vi "Laptop image processing Dev.vi"() -> ()   [LabVIEW 2009]
uses:
  <vilib>/userDefined/High Color/IMAQdx.ctl
  UDP Lib/UDP Network Location.ctl
  TypeDefs/cRIO-EVS Comm/EVS to cRIO UDP packet.ctl
  <vilib>/vision/driver/IMAQdx.llb/IMAQdx Acquisition Mode.ctl
  <vilib>/Platform/TimedLoop/XDataNode/XDataNode.xnode
  <vilib>/Platform/TimedLoop/XDataNode/loadlvalarms.vi
  <vilib>/Platform/TimedLoop/XDataNode/timing_clust.ctl
  <vilib>/Platform/TimedLoop/XDataNode/nitl_modes.ctl
  <vilib>/Platform/TimedLoop/XDataNode/wakeup.ctl
  <vilib>/vision/driver/NI_Vision_Acquisition_Software.lvlib
  <vilib>/Platform/TimedLoop/XDataNode/XDNodeRunTimeDep.lvlib
panel:
  out "Extracted 2":T1(plugin-control) caption="Extracted"
  out "Original 2":T1(plugin-control) caption="Original"
  out "Project:Target Item":refnum<vi>
  out "Original":T1(plugin-control)
  out "Extracted":T1(plugin-control)
  out "Ramp?":bool
  in  "Extraction mode":i32(knob) scale=0.0..2.0
  out "Iteration Duration":i64
  out "Number of ramp regions (left)":i32
  out "Number of ramp regions (right)":i32
  out "Sick array":u16[](array[numeric])
  in  "stop":bool
  out "HB":bool
  in  "IMAQdx Session Left":T2="lcam" caption="Left Session"
  in  "IMAQdx Session Right":T2="rcam" caption="Right Session"
  # "0: Original\n1: Extracted\n2: Masked"
  # "0: Old line extraction\n1: Solid white line (ramp)\n2: LPF"
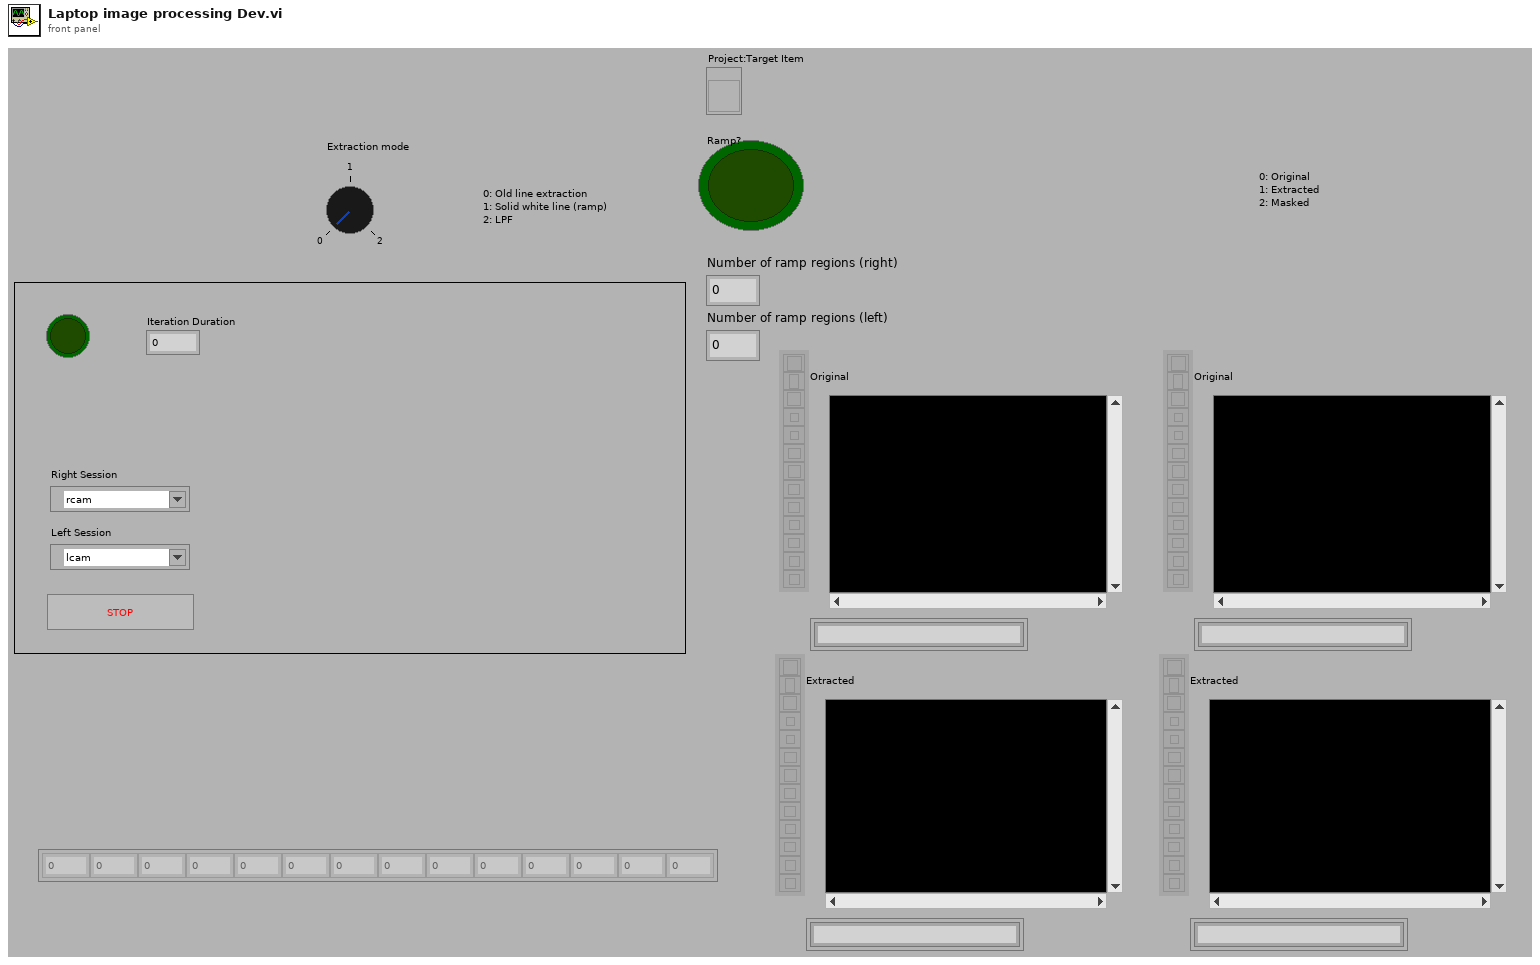
[diagram p1: front panel]
types:
  T1 = typedef "IMAQ Image.ctl" = refnum<image>
  T2 = typedef "IMAQdx.ctl" = refnum<k21>
  T3 = typedef "EVS to cRIO UDP packet.ctl" = cluster{"Camera SICK":u16[], "Camera init":bool}
  T4 = typedef "NI_Vision_Acquisition_Software.lvlib/IMAQdx Acquisition Mode.ctl" = enum32{"One Shot", "Continuous"}
  T5 = typedef "XDNodeRunTimeDep.lvlib/timing_clust.ctl" = cluster{"Expected End [f-1]":u64, "Actual End [f-1]":u64, "Finished Late? [f-1]":bool, "Expected End [i-1]":u64, "Actual End [i-1]":u64, "Finished Late? [i-1]":bool, "Expected Start [i]":u64, "Actual Start [i]":u64, "Expected Start [f]":u64, "Actual Start [f]":u64, "Source Name":string, "Structure Name":string, "Period":i64, "Deadline":i64, "Offset":i64, "Start":i64, "Priority":i32, "Timeout":i32, "Mode":T6, "Wakeup Reason":T7, "Error":errorcluster, "Source Type":string, "Secondary Source Type":string, "Global End Time":u64, "Global Start Time":u64, "Frame Duration":u64, "Iteration Duration":u64, "Assigned CPU":i32, "I/O Scan Engine Mode":u32}
  T6 = typedef "XDNodeRunTimeDep.lvlib/nitl_modes.ctl" = enum32{"No Change", "Process missed periods, maintain original phase", "Discard missed periods, maintain original phase", "Process missed periods, ignore original phase", "Discard missed periods, ignore original phase"}
  T7 = typedef "XDNodeRunTimeDep.lvlib/wakeup.ctl" = enum32{"Normal", "Aborted", "Asynchronous wakeup", "Timing source error", "Timed loop error", "Timeout"}
  T8 = typedef "UDP Network Location.ctl" = cluster{"IP Address":string, "Port":u16}
  T9 = typedef "UDP Base.ctl" = cluster{"UDP Session":refnum<k16>, "UDP Socket Params":T10}
  T10 = typedef "UDP Socket Params.ctl" = cluster{"Local Port":u16, "Read Timeout":i32, "Write Timeout":i32}
  T11 = typedef "Image Type" = u32
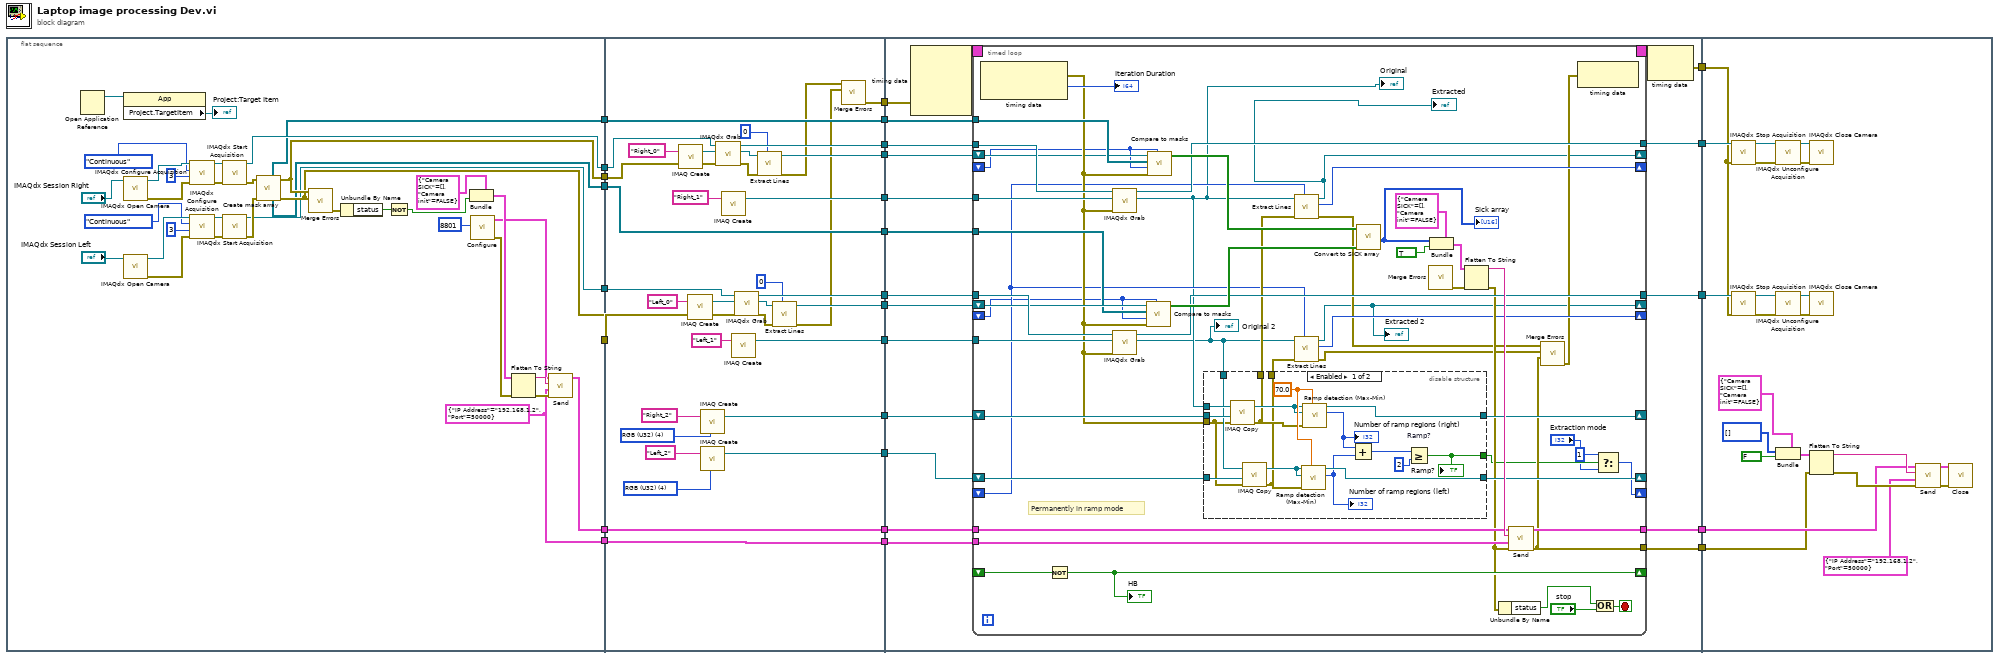
[diagram p0: block diagram]
diagram:
  n1 = flat-sequence {
    tunnel: [w42] -> w26
    tunnel: [w41] -> w25
    tunnel: [w40] -> w24
    tunnel: [w39] -> w23
    tunnel: [w38] -> w16
    tunnel: [w37] -> w14
    tunnel: [w36] -> w13
    tunnel: [w32] -> w5
    tunnel: w26 -> [w91]
    tunnel: w25 -> [w90]
    tunnel: w24 -> [w87]
    tunnel: w23 -> [w86]
    tunnel: [w85] -> w22
    tunnel: [w82] -> w21
    tunnel: [w81] -> w20
    tunnel: [w80] -> w19
    tunnel: [w79] -> w18
    tunnel: [w78] -> w17
    tunnel: w16 -> [w77]
    tunnel: [w77] -> w15
    tunnel: w14 -> [w76]
    tunnel: w13 -> [w75]
    tunnel: [w76] -> w12
    tunnel: [w75] -> w11
    tunnel: [w74] -> w6
    tunnel: w5 -> [w74]
    tunnel: [w71] -> w4
    tunnel: [w70] -> w3
    tunnel: [w67] -> w2
    tunnel: w22 -> [w108]
    tunnel: w21 -> [w107]
    tunnel: w20 -> [w119]
    tunnel: w19 -> [w118]
    tunnel: w18 -> [w117]
    tunnel: w17 -> [w116]
    tunnel: w15 -> [w115]
    tunnel: w12 -> [w114]
    tunnel: w11 -> [w113]
    tunnel: [w112] -> w10
    tunnel: [w111] -> w9
    tunnel: [w110] -> w8
    tunnel: [w109] -> w7
    tunnel: w6 -> [w106]
    tunnel: w4 -> [w103]
    tunnel: w3 -> [w102]
    tunnel: w2 -> [w101]
    tunnel: [w100] -> w1
    tunnel: w10 -> [w213]
    tunnel: w9 -> [w212]
    tunnel: w8 -> [w208]
    tunnel: w7 -> [w207]
    tunnel: w1 -> [w200]
    frame #0 {
      w32 = T8 {"IP Address"="192.168.1.2", "Port"=50000} ("cRIO Network Location")
      n2 = Open Application Reference() -> (3:w28:refnum<vi>)  [unwired: 4 in, 1 out]
      n3 = property class="App"(reference=w28) -> ("Project.TargetItem"=→"Project:Target Item":refnum<vi>)  [unwired: 1 in, 2 out]
      n4 = call <vilib>:"IMAQdx Open Camera.vi"("Session In"="IMAQdx Session Right") -> ("error out"=w61:errorcluster, "Session Out"=w60:T2)  [unwired: 2 in, 7 out]
      n5 = call <vilib>:"IMAQdx Open Camera.vi"("Session In"="IMAQdx Session Left") -> ("error out"=w55:errorcluster, "Session Out"=w56:T2)  [unwired: 2 in, 7 out]
      n6 = call <vilib>:"IMAQdx Configure Acquisition.vi"("error in"=w61, "Number of Buffers"=u32 3, "Continuous?"=IMAQdx_Acquisition_Mode."Continuous", "Session In"=w60) -> ("error out"=w62:errorcluster, "Session Out"=w59:T2)  [unwired: 1 in, 5 out]
      n7 = call <vilib>:"IMAQdx Configure Acquisition.vi"("error in"=w55, "Number of Buffers"=u32 3, "Continuous?"=IMAQdx_Acquisition_Mode."Continuous", "Session In"=w56) -> ("error out"=w54:errorcluster, "Session Out"=w57:T2)  [unwired: 1 in, 5 out]
      n8 = call <vilib>:"IMAQdx Start Acquisition.vi"("error in"=w62, "Session In"=w59) -> ("error out"=w48:errorcluster, "Session Out"=w39:T2)  [unwired: 8 out]
      n9 = call <vilib>:"IMAQdx Start Acquisition.vi"("error in"=w54, "Session In"=w57) -> ("error out"=w47:errorcluster, "Session Out"=w40:T2)  [unwired: 8 out]
      n10 = call "Create mask array.vi"("Left error in"=w47, "Right Error in"=w48) -> ("Left error out"=w41:errorcluster, "Right error out"=w42:errorcluster, "Left Cam Masks"=w36:T1[], "Right Cam Masks"=w37:T1[])  [unwired: 6 in]
      n11 = call <vilib>:"Merge Errors.vi"("error in 2 (no error)"=w41, "error in 1 (no error)"=w42) -> ("error out"=w33:errorcluster)  [unwired: 5 in]
      n12 = Unbundle By Name(w33) -> ("status"=w46:bool)
      n13 = Not(x=w46) -> (.not. x?=w34:bool)
      n14 = Bundle(cluster=T3 {"Camera SICK"=[], "Camera init"=FALSE} ("EVS to cRIO UDP packet"), "Camera init"=w34) -> (w45:T3)  [unwired: 1 in]
      n15 = call "Configure.vi"("Local Port"=u16 8801) -> ("error out"=w29:errorcluster, "UDP Base out"=w30:T9)  [unwired: 9 in]
      n16 = Flatten To String(anything=w45, error in (no error)=w29) -> (data string=w44:string, error out=w43:errorcluster)  [unwired: 2 in, 1 out]
      n17 = call "Send.vi"("error in (no error)"=w43, "Destination Location"=w32, "Send Data"=w44, "UDP Base in"=w30) -> ("UDP Base out"=w38:T9)  [unwired: 5 in, 2 out]
    }
    frame #1 {
      w65 = T11 4 items=["Grayscale (U8)", "Grayscale (I16)", "Grayscale (SGL)", "Complex (CSG)", "RGB (U32)", "HSL (U32)", "RGB (U64)", "Grayscale (U16)"] ("Image Type")
      w66 = T11 4 items=["Grayscale (U8)", "Grayscale (I16)", "Grayscale (SGL)", "Complex (CSG)", "RGB (U32)", "HSL (U32)", "RGB (U64)", "Grayscale (U16)"] ("Image Type")
      n18 = call "IMAQ Create"("Image Name"="Right_0", "error in (no error)"=w91) -> ("New Image"=w93:T1, "error out"=w92:errorcluster)  [unwired: 3 in]
      n19 = call "IMAQ Create"("Image Name"="Left_0", "error in (no error)"=w90) -> ("New Image"=w95:T1, "error out"=w94:errorcluster)  [unwired: 3 in]
      n20 = call "IMAQ Create"("Image Name"="Right_2", "Image Type"=w66) -> ("New Image"=w71:T1)  [unwired: 3 in, 1 out]
      n21 = call "IMAQ Create"("Image Name"="Left_2", "Image Type"=w65) -> ("New Image"=w70:T1)  [unwired: 3 in, 1 out]
      n22 = call <vilib>:"IMAQdx Grab.vi"("error in"=w92, "Image In"=w93, "Session In"=w86) -> ("error out"=w99:errorcluster, "Image Out"=w96:T1, "Session Out"=w81:T2)  [unwired: 5 in, 1 out]
      n23 = call "IMAQ Create"("Image Name"="Right_1") -> ("New Image"=w85:T1)  [unwired: 4 in, 1 out]
      n24 = call "IMAQ Create"("Image Name"="Left_1") -> ("New Image"=w82:T1)  [unwired: 4 in, 1 out]
      n25 = call <vilib>:"IMAQdx Grab.vi"("error in"=w94, "Image In"=w95, "Session In"=w87) -> ("error out"=w98:errorcluster, "Image Out"=w97:T1, "Session Out"=w80:T2)  [unwired: 5 in, 1 out]
      n26 = call "Extract Lines.vi"("Extraction mode"=0, "error in (no error)"=w99, "Image Src"=w96) -> ("error out"=w69:errorcluster, "Image Out"=w79:T1)  [unwired: 6 in, 1 out]
      n27 = call "Extract Lines.vi"("Extraction mode"=0, "error in (no error)"=w98, "Image Src"=w97) -> ("error out"=w68:errorcluster, "Image Out"=w78:T1)  [unwired: 6 in, 1 out]
      n28 = call <vilib>:"Merge Errors.vi"("error in 2 (no error)"=w68, "error in 1 (no error)"=w69) -> ("error out"=w67:errorcluster)  [unwired: 5 in]
    }
    frame #2 {
      n29 = node-c288(w101) -> (w105:T5)  [unwired: 3 in]
      n30 = timed-loop {
        tunnel: w119 -> [w171]
        tunnel: w118 -> [w170]
        shift-right: [w125] -> _
        shift-left: w117 -> [w126]
        shift-right: [w120] -> _
        shift-left: w116 -> [w169]
        shift-right: [w142] -> _
        shift-left: _ -> [w122]
        shift-right: [w143] -> _
        shift-left: _ -> [w123]
        tunnel: w115 -> [w165]
        tunnel: [w164] -> w110
        tunnel: [w136] -> w109
        tunnel: w114 -> [w163]
        tunnel: w113 -> [w162]
        tunnel: [w161] -> w111
        tunnel: [w160] -> w112
        tunnel: w108 -> [w159]
        tunnel: w107 -> [w158]
        tunnel: w106 -> [w153]
        shift-right: [w152] -> _
        shift-left: _ -> [w151]
        timing: w105 -> [_]
        timing-out: [_] -> w104
        shift-right: [w149] -> _
        shift-left: w103 -> [w141]
        shift-right: [w148] -> _
        shift-left: w102 -> [w140]
        shift-right: [w127] -> _
        shift-left: _ -> [w131]
        stop <- w147 stop-if-true
        # "Permanently in ramp mode"
        n31 = node-c288() -> (w139:errorcluster, →"Iteration Duration":i64)  [unwired: 1 in]
        n32 = Not(x=w151) -> (.not. x?=w152:bool)
        "HB" <- w152
        n33 = call <vilib>:"IMAQdx Grab.vi"("error in"=w139, "Image In"=w159, "Session In"=w171) -> ("Image Out"=w124:T1, "Session Out"=w161:T2)  [unwired: 5 in, 2 out]
        "Original" <- w124
        n34 = call <vilib>:"IMAQdx Grab.vi"("error in"=w139, "Image In"=w158, "Session In"=w170) -> ("Image Out"=w121:T1, "Session Out"=w160:T2)  [unwired: 5 in, 2 out]
        "Original 2" <- w121
        n35 = call "Compare to masks.vi"("Number of Particles1"=w122, "error in (no error)"=w139, "Number of Particles"=w122, "Mask array"=w162, "Image Src"=w169) -> ("Marked Regions"=w167:bool[])  [unwired: 5 in, 1 out]
        n36 = call "Compare to masks.vi"("Number of Particles1"=w123, "error in (no error)"=w139, "Number of Particles"=w123, "Mask array"=w163, "Image Src"=w126) -> ("Marked Regions"=w168:bool[])  [unwired: 5 in, 1 out]
        n37 = disable-structure shown="Enabled" {
          disable-tunnel: [w188 _] -> w149
          disable-tunnel: [w187 _] -> w148
          disable-tunnel: [w181 _] -> w130
          disable-tunnel: w141 -> [w180 _]
          disable-tunnel: w124 -> [w179 _]
          disable-tunnel: w121 -> [w178 _]
          disable-tunnel: w140 -> [w177 _]
          disable-tunnel: w139 -> [w176 _]
          disable-tunnel: [w173 _] -> w133
          disable-tunnel: [w172 _] -> w132
          frame #0 {
            w186 = sgl 70.0 ("Tolerance")
            n38 = call "IMAQ Copy"("error in (no error)"=w176, "Image Dst"=w180, "Image Src"=w179) -> ("error out"=w173:errorcluster, "Image Dst Out"=w175:T1)  [unwired: 3 in]
            n39 = call "IMAQ Copy"("error in (no error)"=w176, "Image Dst"=w177, "Image Src"=w178) -> ("error out"=w172:errorcluster, "Image Dst Out"=w174:T1)  [unwired: 3 in]
            n40 = call "Ramp detection (Max-Min).vi"("Tolerance"=w186, "error in (no error)"=w172, "Image Dst"=w174, "Image Src"=w174) -> ("Number of ramp regions"=w184:i32, "Image Out"=w187:T1)  [unwired: 5 in, 1 out]
            "Number of ramp regions (left)" <- w184
            n41 = call "Ramp detection (Max-Min).vi"("Tolerance"=w186, "error in (no error)"=w173, "Image Dst"=w175, "Image Src"=w175) -> ("Number of ramp regions"=w185:i32, "Image Out"=w188:T1)  [unwired: 5 in, 1 out]
            "Number of ramp regions (right)" <- w185
            n42 = Add(x=w185, y=w184) -> (x+y=w183:i32)
            n43 = Greater Or Equal? "Ramp?"(x=w183, y=2) -> (x >= y?=w181:bool)
            "Ramp?" <- w181
          }
          frame #1 {
          }
        }
        n44 = call "Extract Lines.vi"("Extraction mode"=w131, "error in (no error)"=w133, "Image Src"=w124) -> ("error out"=w135:errorcluster, "Number of Particles1"=w143:i32, "Image Out"=w125:T1)  [unwired: 6 in]
        "Extracted" <- w125
        n45 = call "Extract Lines.vi"("Extraction mode"=w131, "error in (no error)"=w132, "Image Src"=w121) -> ("error out"=w134:errorcluster, "Number of Particles1"=w142:i32, "Image Out"=w120:T1)  [unwired: 6 in]
        "Extracted 2" <- w120
        n46 = call "Convert to SICK array.vi"("Left Regions"=w167, "Right Regions"=w168) -> ("Sick array"=w138:u16[])  [unwired: 9 in]
        "Sick array" <- w138
        n47 = call <vilib>:"Merge Errors.vi"() -> ("error out"=w145:errorcluster)  [unwired: 7 in]
        n48 = Bundle(cluster=T3 {"Camera SICK"=[], "Camera init"=FALSE} ("EVS to cRIO UDP packet"), "Camera SICK"=w138, "Camera init"=TRUE) -> (w154:T3)
        n49 = Flatten To String(anything=w154, error in (no error)=w145) -> (data string=w166:string, error out=w144:errorcluster)  [unwired: 2 in, 1 out]
        n50 = Unbundle By Name(w144) -> ("status"=w157:bool)
        n51 = call "Send.vi"("error in (no error)"=w144, "Destination Location"=w153, "Send Data"=w166, "UDP Base in"=w165) -> ("error out"=w136:errorcluster, "UDP Base out"=w164:T9)  [unwired: 5 in, 1 out]
        n52 = call <vilib>:"Merge Errors.vi"("error in 3 (no error)"=w136, "error in 2 (no error)"=w134, "error in 1 (no error)"=w135) -> ("error out"=w137:errorcluster)  [unwired: 4 in]
        n53 = node-c288(w137) -> ()  [unwired: 1 out]
        n54 = Or(x=w157, y="stop") -> (x .or. y?=w147:bool)
        n55 = Select(t=1, s=w130, f="Extraction mode") -> (s? t:f=w127:i32)
      }
      n56 = node-c288(w104) -> (w100:errorcluster)
    }
    frame #3 {
      n57 = call <vilib>:"IMAQdx Stop Acquisition.vi"("error in"=w200, "Session In"=w212) -> ("error out"=w219:errorcluster, "Session Out"=w218:T2)  [unwired: 8 out]
      n58 = call <vilib>:"IMAQdx Stop Acquisition.vi"("error in"=w200, "Session In"=w213) -> ("error out"=w215:errorcluster, "Session Out"=w214:T2)  [unwired: 8 out]
      n59 = call <vilib>:"IMAQdx Unconfigure Acquisition.vi"("error in"=w219, "Session In"=w218) -> ("error out"=w220:errorcluster, "Session Out"=w221:T2)  [unwired: 8 out]
      n60 = call <vilib>:"IMAQdx Unconfigure Acquisition.vi"("error in"=w215, "Session In"=w214) -> ("error out"=w216:errorcluster, "Session Out"=w217:T2)  [unwired: 8 out]
      n61 = Bundle(cluster=T3 {"Camera SICK"=[], "Camera init"=FALSE} ("EVS to cRIO UDP packet"), "Camera SICK"=u16[] [], "Camera init"=FALSE) -> (w202:T3)
      n62 = call <vilib>:"IMAQdx Close Camera.vi"("error in"=w220, "Session In"=w221) -> ()  [unwired: 10 out]
      n63 = call <vilib>:"IMAQdx Close Camera.vi"("error in"=w216, "Session In"=w217) -> ()  [unwired: 10 out]
      n64 = Flatten To String(anything=w202, error in (no error)=w207) -> (data string=w211:string, error out=w210:errorcluster)  [unwired: 2 in, 1 out]
      n65 = call "Send.vi"("error in (no error)"=w210, "Destination Location"=T8 {"IP Address"="192.168.1.2", "Port"=50000}, "Send Data"=w211, "UDP Base in"=w208) -> ("error out"=w205:errorcluster, "UDP Base out"=w206:T9)  [unwired: 5 in, 1 out]
      n66 = call "Close.vi"("error in (no error)"=w205, "Cluster of class private data"=w206) -> ()  [unwired: 9 in, 1 out]
    }
  }
